vi "Trigger Circuitry (Advanced).vi"(6 "State Machine State":T2, 7 "Trigger Type":T3(ring)=enum."Software Trigger", 9 "Analog Trigger Setup":T1, 10 "Digital Trigger Value":u8, 11 "Software Trigger from Host":bool) -> (0 "Trigger Info":cluster{"Trigger":bool, "Trig Offset":u8}, 2 "Trigger Out":bool, 3 "Analog Arm Trig":bool)   [LabVIEW 2011]
uses:
  <instrlib>/FlexRIO/Libraries/Acquisition Engine/FPGA/Interface/acqEngineStates v1.ctl
  <vilib>/rvi/FXPMathLib/basic elements/FxpDiscreteDelay/XNode/nifxpmath_DiscreteDelay.xnode
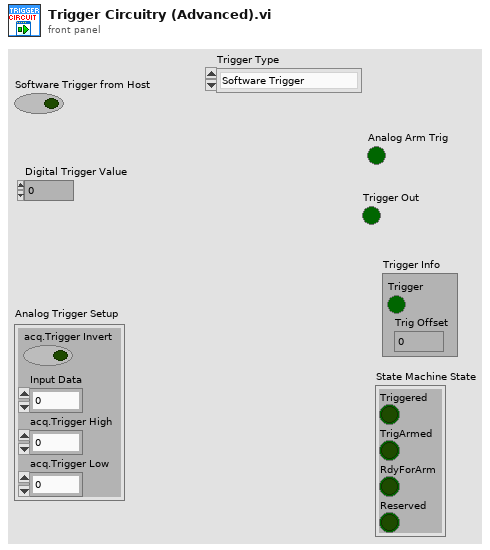
[diagram p1: front panel]
types:
  T1 = cluster{"acq.Trigger Invert":bool, "Input Data":i16, "acq.Trigger High":i16, "acq.Trigger Low":i16}
  T2 = typedef "acqEngineStates v1.ctl" = cluster{"Triggered":bool, "TrigArmed":bool, "RdyForArm":bool, "Reserved":bool}
  T3 = enum8{"Immediate Trigger", "Software Trigger", "External Digital Trigger", "Analog Trigger"}
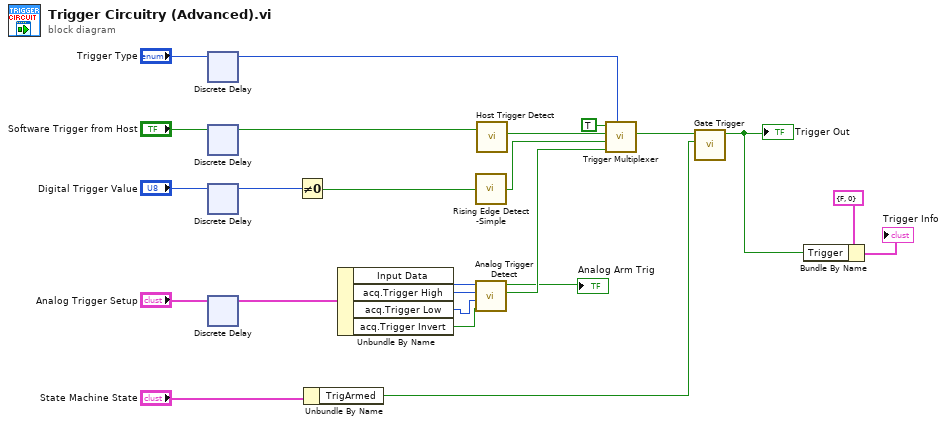
[diagram p0: block diagram]
diagram:
  n1 = xnode "Discrete Delay"("D"="Trigger Type") -> ("Q"=w4:T3)
  n2 = xnode "Discrete Delay"("D"="Software Trigger from Host") -> ("Q"=w3:bool)
  n3 = xnode "Discrete Delay"("D"="Digital Trigger Value") -> ("Q"=w2:u8)
  n4 = xnode "Discrete Delay"("D"="Analog Trigger Setup") -> ("Q"=w1:T1)
  n5 = Not Equal To 0?(x=w2) -> (x != 0?=w6:bool)
  n6 = Unbundle By Name("State Machine State") -> ("TrigArmed"=w17:bool)
  n7 = Unbundle By Name(w1) -> ("Input Data"=w14:i16, "acq.Trigger High"=w13:i16, "acq.Trigger Low"=w12:i16, "acq.Trigger Invert"=w11:bool)
  n8 = call <userlib>:"Rising Edge Detect -Simple.vi"("signal"=w6) -> ("edge detected"=w5:bool)  [unwired: 14 in]
  n9 = call <userlib>:"Analog Trigger Detect.vi"("acq.Trigger Invert"=w11, "acq.Trigger High"=w12, "acq.Trigger Low"=w13, "Input Data"=w14) -> ("Analog Trigger Detect"=w21:bool, "Analog Arm Trig"=→"Analog Arm Trig":bool)  [unwired: 6 in]
  n10 = call <userlib>:"Host Trigger Detect.vi"("Software Trigger from Host"=w3) -> ("Host Rising Edge Detect"=w22:bool)  [unwired: 10 in]
  n11 = call <userlib>:"Trigger Multiplexer.vi"("Trigger Type"=w4, "Analog Trigger"=w21, "Digital Trigger"=w5, "Software Trigger"=w22, "Immediate Trigger"=TRUE) -> ("Trigger Out"=w18:bool)  [unwired: 6 in]
  n12 = call <userlib>:"Gate Trigger.vi"("Gate Signal'"=w17, "Trigger"=w18) -> ("Ref Trig"=w8:bool)  [unwired: 9 in]
  "Trigger Out" <- w8
  n13 = Bundle By Name(cluster=cluster{"Trigger":bool, "Trig Offset":u8} {"Trigger"=FALSE, "Trig Offset"=0} ("Trigger Info"), "Trigger"=w8) -> (→"Trigger Info":cluster{"Trigger":bool, "Trig Offset":u8})
